vi "Init Scintilla.vi"(8 "error in (no error)":errorcluster, 11 "LF2R IDE in":refnum<class "Main Panel.lvclass">) -> (0 "error out":errorcluster, 3 "LF2R IDE out":refnum<class "Main Panel.lvclass">)   [LabVIEW 2018, in "Main Panel.lvlib" / "Main Panel.lvclass"]
uses:
  Main Panel.lvclass
  D:/project/hobby/LabVIEW/LF2R/LabVIEW/Source/ScintillaNET/dll/ScintillaNET.dll
  ScintillaNET/dll/ScintillaNET.dll
  Main Panel.lvclass/Main Panel.ctl
  ScintillaNET/ScintillaNET.lvclass
  Frame Analizer/Data Parser.lvclass
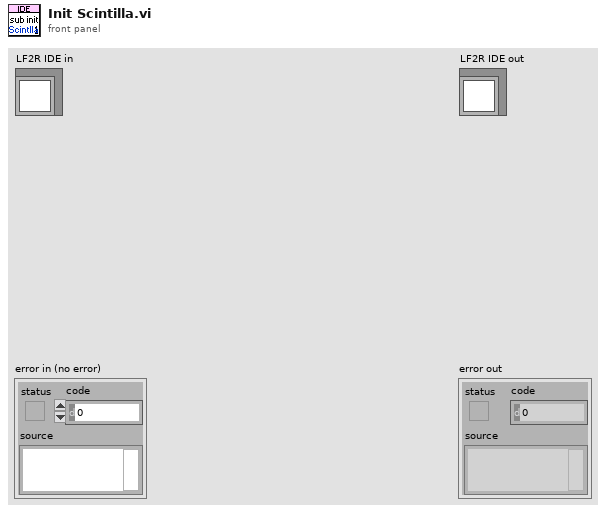
[diagram p1: front panel]
types:
  T1 = cluster{"Color":u32, "Bold":bool, "Italic":bool, "FillLine":bool}
  T2 = cluster{"Type":i32, "Width":i32, "Sensitive":bool, "Mask":u32, "Cursor":i32}
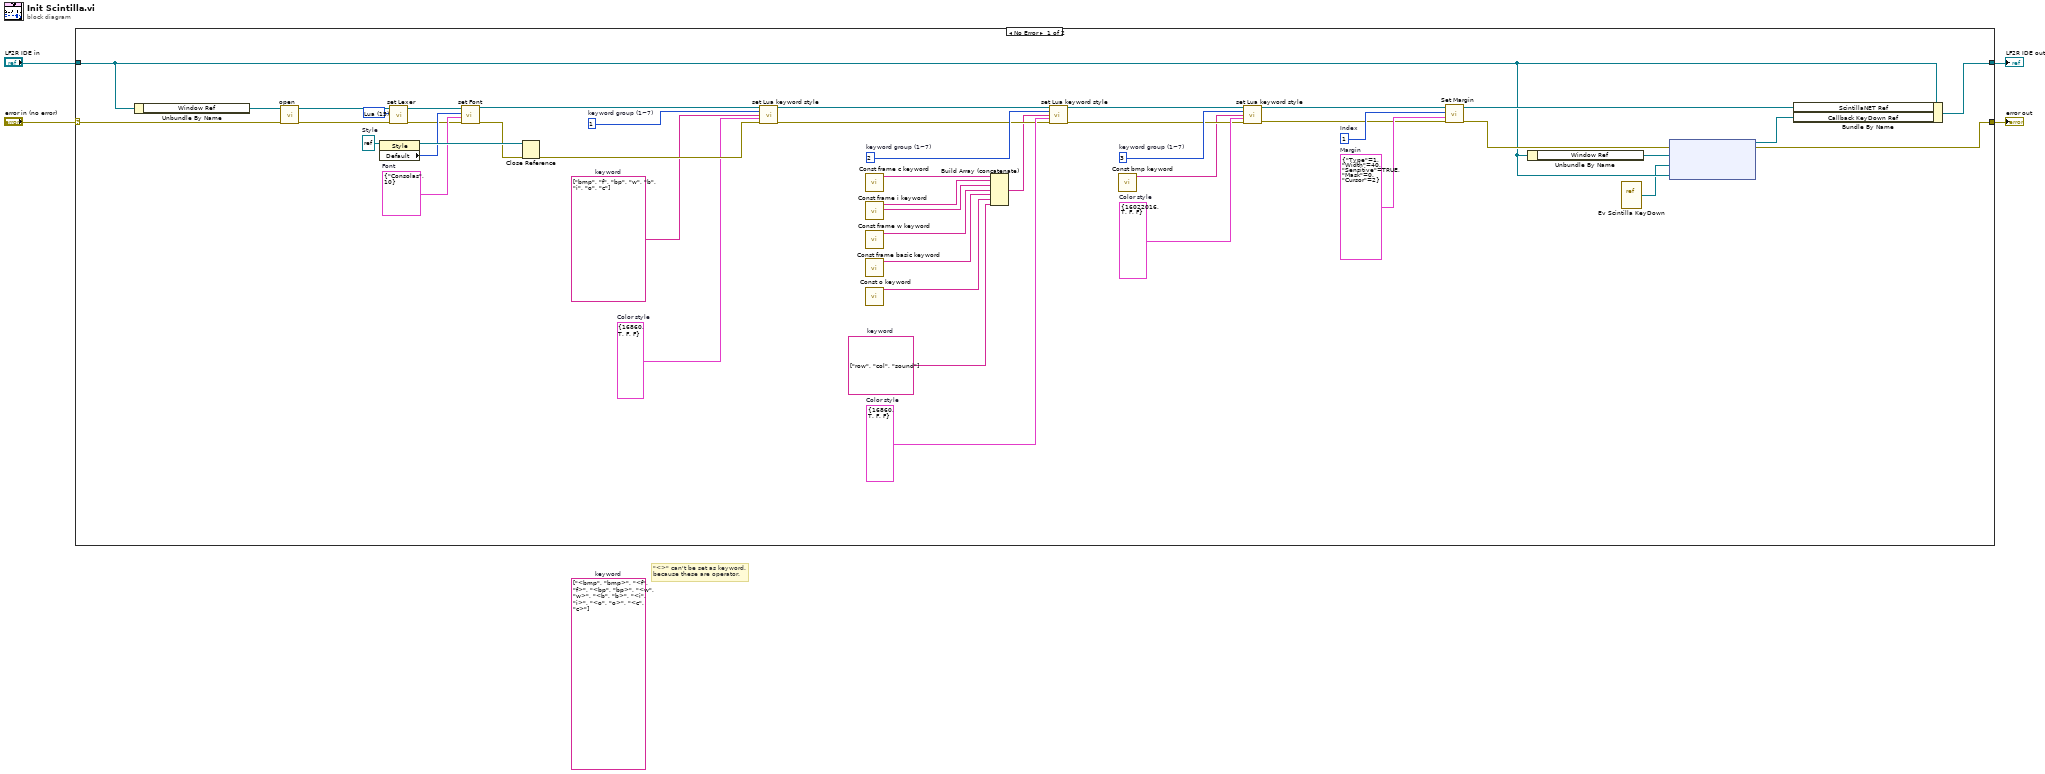
[diagram p0: block diagram]
diagram:
  (unwired) string[] ["<bmp", "bmp>", "<f", "f>", "<bp", "bp>", "<w", "w>", "<b", "b>", "<i", "i>", "<o", "o>", "<c", "c>"]  # keyword
  # "\"<>\" can't be set as keyword.\nbecause these are operator."
  n1 = case shown="No Error" "error in (no error)" {
    selector: "error in (no error)" -> [w46 w52]
    tunnel: [w8 w52] -> w3
    tunnel: [w33 w51] -> w1
    tunnel: "LF2R IDE in" -> [w7 w51]
    frame No Error {
      w18 = T1 {"Color"=16022016, "Bold"=TRUE, "Italic"=FALSE, "FillLine"=FALSE}  # Color style
      w19 = 3  # keyword group (1~7)
      w20 = string[] ["row", "col", "sound"]  # keyword
      w30 = T1 {"Color"=16860, "Bold"=TRUE, "Italic"=FALSE, "FillLine"=FALSE}  # Color style
      w29 = 2  # keyword group (1~7)
      w31 = T2 {"Type"=1, "Width"=40, "Sensitive"=TRUE, "Mask"=0, "Cursor"=2}  # Margin
      w32 = 1  # Index
      w34 = T1 {"Color"=16860, "Bold"=TRUE, "Italic"=FALSE, "FillLine"=FALSE}  # Color style
      w35 = string[] ["bmp", "f", "bp", "w", "b", "i", "o", "c"]  # keyword
      w36 = 1  # keyword group (1~7)
      w41 = cluster{"Font":string, "Size":i32} {"Font"="Consolas", "Size"=10}  # Font
      w45 = refnum<k24> refnum  # Style
      w47 = 15 items=["Container"=0, "Null"=1, "Python"=2, "Cpp"=3, "Html"=4, "Xml"=5, "Perl"=6, "Sql"=7, "Vb"=8, "Properties"=9, "Batch"=12, "Lua"=15, "Pascal"=18, "Ada"=20, "Lisp"=21, "Ruby"=22, "VbScript"=28, "Asm"=34, "Fortran"=36, "Css"=38, "Verilog"=56, "BlitzBasic"=66, "PureBasic"=67, "PhpScript"=69, "Smalltalk"=72, "FreeBasic"=75, "R"=86, "PowerShell"=88, "Markdown"=98, "Json"=120] ("Lexer")
      n2 = Unbundle By Name(w7) -> ("Window Ref"=w50:refnum<k24>)
      n3 = call "open.vi"("error in (no error)"=w46, "Scintilla window ref"=w50) -> ("error out"=w48:errorcluster, "ScintillaNET out"=w49:refnum<class "ScintillaNET.lvclass">)  [unwired: 8 in]
      n4 = property class="Style"(reference=w45) -> (reference out=w44:refnum<k24>, "Default"=w42:i32)  [unwired: 1 in, 1 out]
      n5 = call "set Lexer.vi"("error in (no error)"=w48, "Lexer"=w47, "ScintillaNET in"=w49) -> ("error out"=w39:errorcluster, "ScintillaNET out"=w40:refnum<class "ScintillaNET.lvclass">)  [unwired: 7 in]
      n6 = call "set Font.vi"("error in (no error)"=w39, "Font"=w41, "Style index"=w42, "ScintillaNET in"=w40) -> ("error out"=w43:errorcluster, "ScintillaNET out"=w38:refnum<class "ScintillaNET.lvclass">)  [unwired: 6 in]
      n7 = Close Reference(reference=w44, error in (no error)=w43) -> (error out=w37:errorcluster)
      n8 = call "set Lua keyword style.vi"("ScintillaNET in"=w38, "keyword group (1~7)"=w36, "keyword"=w35, "Color style"=w34, "error in (no error)"=w37) -> ("ScintillaNET out"=w28:refnum<class "ScintillaNET.lvclass">, "error out"=w27:errorcluster)  [unwired: 9 in]
      n9 = call "Const frame c keyword.vi"() -> ("Const frame c keyword"=w26:string[])  [unwired: 11 in]
      n10 = call "Const frame i keyword.vi"() -> ("Const frame i keyword 2"=w24:string[], "Const frame i keyword"=w25:string[])  [unwired: 10 in]
      n11 = call "Const frame w keyword.vi"() -> ("Const frame w keyword"=w23:string[])  [unwired: 11 in]
      n12 = call "Const frame basic keyword.vi"() -> ("Const frame basic keyword"=w22:string[])  [unwired: 11 in]
      n13 = call "Const o keyword.vi"() -> ("Const o keyword"=w12:string[])  [unwired: 11 in]
      n14 = Build Array (concatenate)(w26, w25, w24, w23, w22, w12, w20) -> (w21:string[])
      n15 = call "set Lua keyword style.vi"("ScintillaNET in"=w28, "keyword group (1~7)"=w29, "keyword"=w21, "Color style"=w30, "error in (no error)"=w27) -> ("ScintillaNET out"=w17:refnum<class "ScintillaNET.lvclass">, "error out"=w16:errorcluster)  [unwired: 9 in]
      n16 = call "Const bmp keyword.vi"() -> ("Const bmp keyword"=w13:string[])  [unwired: 11 in]
      n17 = call "set Lua keyword style.vi"("ScintillaNET in"=w17, "keyword group (1~7)"=w19, "keyword"=w13, "Color style"=w18, "error in (no error)"=w16) -> ("ScintillaNET out"=w15:refnum<class "ScintillaNET.lvclass">, "error out"=w14:errorcluster)  [unwired: 9 in]
      n18 = call "Set Margin.vi"("error in (no error)"=w14, "Margin"=w31, "Index"=w32, "ScintillaNET in"=w15) -> ("error out"=w10:errorcluster, "ScintillaNET out"=w11:refnum<class "ScintillaNET.lvclass">)  [unwired: 6 in]
      n19 = Unbundle By Name(w7) -> ("Window Ref"=w6:refnum<k24>)
      n20 = vi-ref "Ev Scintilla KeyDown.vi"() -> ("vi reference"=w5:refnum<vi>)
      n21 = node(w10, w6, w5, w7) -> (w9:refnum<k27>, w8:errorcluster)  [unwired: 1 in]
      n22 = Bundle By Name(cluster=w7, "ScintillaNET Ref"=w11, "Callback KeyDown Ref"=w9) -> (w33:refnum<class "Main Panel.lvclass">)
    }
    frame Error {
    }
  }
  "error out" <- w3
  "LF2R IDE out" <- w1
